vi "Close.vi"(11 "Channel Data In":T1) -> (3 "Channel Data":T1)   [LabVIEW 2020, in "Flex.lvlib"]
uses:
  Flex.lvlib
  Channel Data.ctl
  Element Info.ctl
  Element.ctl
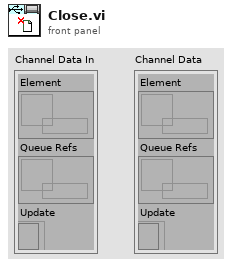
[diagram p1: front panel]
types:
  T1 = typedef "Flex.lvlib/Channel Data.ctl" = cluster{"Element":refnum<data-value>, "Queue Refs":refnum<data-value>, "Update":refnum<k4>}
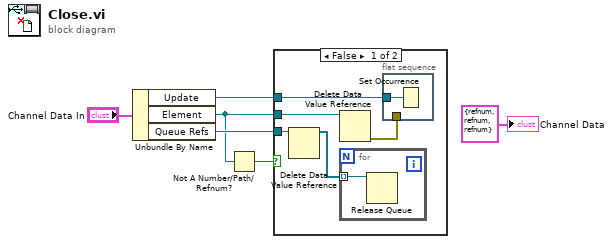
[diagram p0: block diagram]
diagram:
  n1 = Unbundle By Name("Channel Data In") -> ("Update"=w3:refnum<k4>, "Element"=w2:refnum<data-value>, "Queue Refs"=w4:refnum<data-value>)
  n2 = Not A Number/Path/Refnum?(number/path/refnum=w2) -> (NaN/Path/Refnum?=w1:bool)
  n3 = case shown="False" w1 {
    tunnel: w4 -> [w11 _]
    tunnel: w3 -> [w9 _]
    tunnel: w2 -> [w7 _]
    frame False {
      n4 = Delete Data Value Reference(data value reference=w11) -> (data value=w10:refnum<queue>[])  [unwired: 1 in, 1 out]
      n5 = Delete Data Value Reference(data value reference=w7) -> (error out=w8:errorcluster)  [unwired: 1 in, 1 out]
      n6 = for {
        tunnel: w10 -> [w13] mode=indexing
        n7 = Release Queue(queue=w13) -> ()  [unwired: 2 in, 3 out]
      }
      n8 = flat-sequence {
        tunnel: w9 -> [w12]
        tunnel: w8 -> [_]
        frame #0 {
          n9 = Set Occurrence(w12) -> ()
        }
      }
    }
    frame True {
      # "Already closed"
    }
  }
  "Channel Data" <- T1 {"Element"=refnum, "Queue Refs"=refnum, "Update"=refnum} ("Channel Data")
